vi "Decimate Correction Array (SubVI).vi"(7 "Decimation":dbl, 11 "Compensation In (%)":cluster{dbl[], dbl[]}) -> (3 "Compensation Out (%)":cluster{"xi used":dbl[], "yi":dbl[]})   [LabVIEW 2016]
uses:
  <vilib>/gmath/NI_Gmath.lvlib
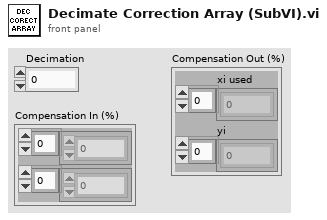
[diagram p1: front panel]
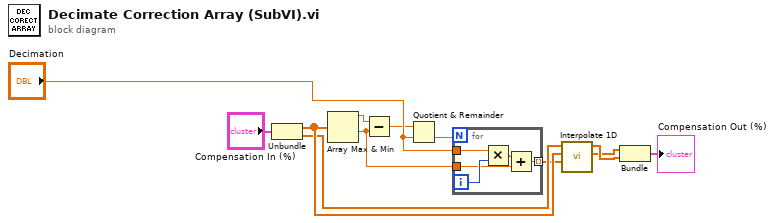
[diagram p0: block diagram]
diagram:
  n1 = Unbundle("Compensation In (%)") -> (w9:dbl[], w8:dbl[])
  n2 = Array Max & Min(array=w9) -> (max value=w1:dbl, min value=w3:dbl)  [unwired: 2 out]
  n3 = Subtract(x=w1, y=w3) -> (x-y=w2:dbl)
  n4 = Quotient & Remainder(x=w2, y="Decimation") -> (floor(x/y)=w5:dbl)  [unwired: 1 out]
  n5 = for {
    N: w5 -> [_]
    tunnel: "Decimation" -> [w15]
    tunnel: w3 -> [w14]
    tunnel: [w13] -> w7 mode=indexing
    i -> [w17]
    n6 = Multiply(x=w15, y=w17) -> (x*y=w16:dbl)
    n7 = Add(x=w16, y=w14) -> (x+y=w13:dbl)
  }
  n8 = call <vilib>:"Interpolate 1D.vi"("xi"=w7, "X"=w9, "Y"=w8) -> ("xi used"=w10:dbl[], "yi"=w11:dbl[])  [unwired: 6 in, 1 out]
  n9 = Bundle("xi used"=w10, "yi"=w11) -> (→"Compensation Out (%)":cluster{"xi used":dbl[], "yi":dbl[]})  [unwired: 1 in]
